vi "Get DataPoint Example.vi"() -> ()   [LabVIEW 2019]
uses:
  C:/Users/tim/Documents/kSAComm LabView Sample/kSACommInterface.dll
  kSACommInterface.dll
panel:
  out "LastError":string
  out "Connect Status":bool
  in  "IP":string="192.168.0.169"
  out "Data Point Value":string
  in  "Exit":bool
  in  "Get Data Point":bool
  # "This VI will connect with the kSA application running on the PC with the following IP Address:"
  # "Pressing this button will initiate a read of the DataPoint ColumnID from the kSA application."
  # "Pressing \"Exit\" will cleanly disconnect from the kSA application and quit the VI."
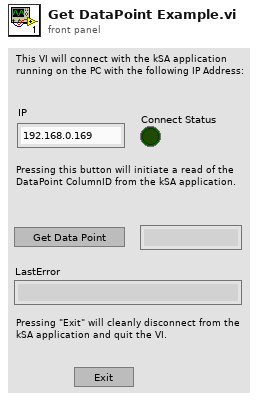
[diagram p1: front panel]
types:
  T1 = cluster{"name":string, "id":u32, "precision":i32}
  T2 = cluster{"name":string, "id":u32, "precision":i32}[]
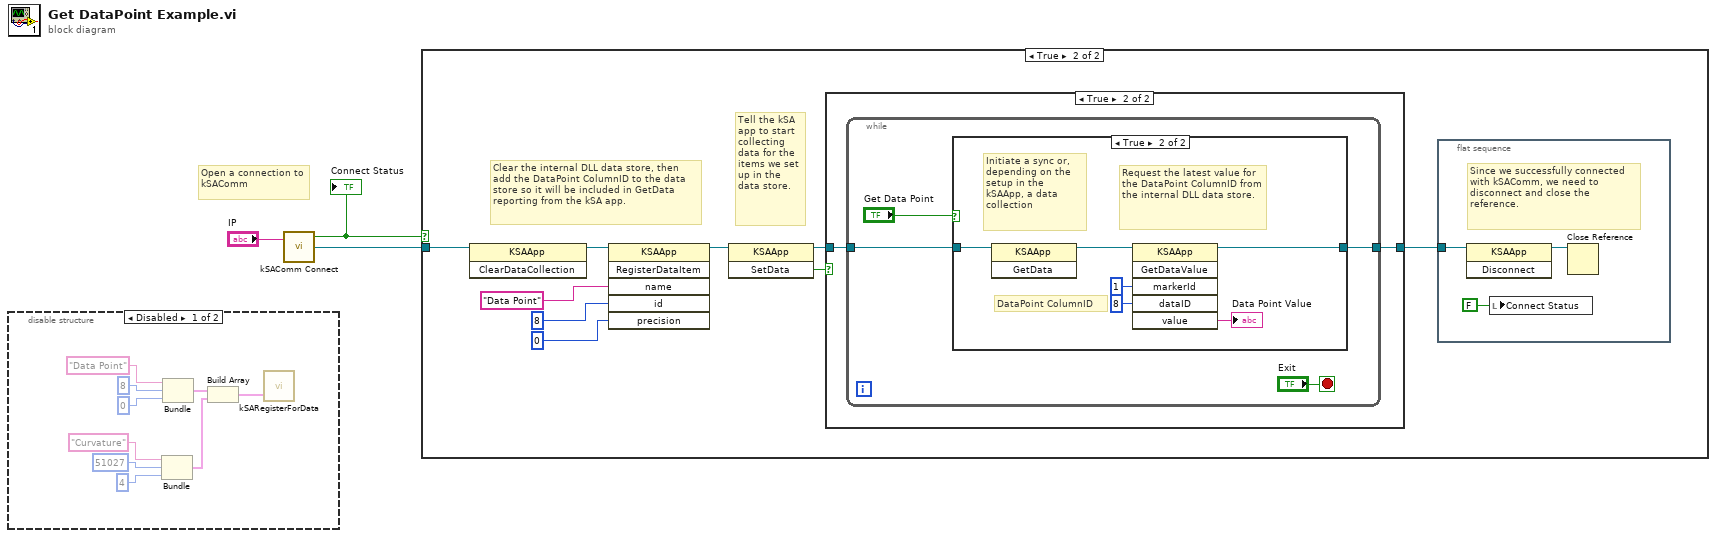
[diagram p0: block diagram]
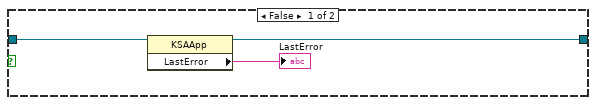
[diagram p4: hidden frame]
diagram:
  # "Open a connection to kSAComm"
  n1 = disable-structure shown="Disabled" {
    frame Disabled {
      n2 = Bundle("name"="Curvature", "id"=u32 51027, "precision"=4) -> (w4:T1)  [unwired: 1 in]
      n3 = Bundle("name"="Data Point", "id"=u32 8, "precision"=0) -> (w9:T1)  [unwired: 1 in]
      n4 = Build Array(w9, w4) -> (w8:T2)
      n5 = call "kSARegisterForData.vi"("Data Definitions"=w8) -> ()  [unwired: 1 in, 2 out]
    }
    frame Enabled {
    }
  }
  n6 = call "kSAComm Connect.vi"("IP Address"="IP") -> ("Connect"=w3:bool, "kSAComm ref out"=w1:refnum<k24>)  [unwired: 2 in]
  "Connect Status" <- w3
  n7 = case shown="True" w3 {
    tunnel: w1 -> [_ w14]
    frame False {
    }
    frame True {
      # "Tell the kSA app to start collecting data for the items we set up in the data store."
      # "Clear the internal DLL data store, then add the DataPoint ColumnID to the data store so it will be included in GetData reporting from the kSA app."
      n8 = invoke class="KSAApp" method="ClearDataCollection"(reference=w14) -> (reference out=w20:refnum<k24>)  [unwired: 2 in, 2 out]
      n9 = invoke class="KSAApp" method="RegisterDataItem"(reference=w20, "name"="Data Point", "id"=u32 8, "precision"=0) -> (reference out=w19:refnum<k24>)  [unwired: 2 in, 5 out]
      n10 = invoke class="KSAApp" method="SetData"(reference=w19) -> (reference out=w15:refnum<k24>, "SetData"=w13:bool)  [unwired: 2 in, 1 out]
      n11 = case shown="True" w13 {
        tunnel: [w22 w25] -> w21
        tunnel: w15 -> [w24 w26]
        frame False {
          n12 = property class="KSAApp"(reference=w24) -> (reference out=w22:refnum<k24>, "LastError"=→"LastError":string)  [unwired: 1 in, 1 out]
        }
        frame True {
          n13 = while {
            tunnel: w26 -> [w29]
            tunnel: [w28] -> w25
            stop <- "Exit" stop-if-true
            n14 = case shown="True" "Get Data Point" {
              tunnel: w29 -> [w31 w37]
              tunnel: [w31 w33] -> w28
              frame False {
              }
              frame True {
                # "Request the latest value for the DataPoint ColumnID from the internal DLL data store."
                # "Initiate a sync or, depending on the setup in the kSAApp, a data collection"
                # "DataPoint ColumnID"
                n15 = invoke class="KSAApp" method="GetData"(reference=w37) -> (reference out=w32:refnum<k24>)  [unwired: 2 in, 2 out]
                n16 = invoke class="KSAApp" method="GetDataValue"(reference=w32, "markerId"=u32 1, "dataID"=u32 8) -> (reference out=w33:refnum<k24>, "value"=→"Data Point Value":string)  [unwired: 3 in, 4 out]
              }
            }
          }
        }
      }
      n17 = flat-sequence {
        tunnel: w21 -> [w39]
        frame #0 {
          # "Since we successfully connected with kSAComm, we need to disconnect and close the reference."
          n18 = invoke class="KSAApp" method="Disconnect"(reference=w39) -> (reference out=w40:refnum<k24>)  [unwired: 2 in, 2 out]
          n19 = local write "Connect Status"(FALSE ("Connect")) -> ()
          n20 = Close Reference(reference=w40) -> ()  [unwired: 1 in, 1 out]
        }
      }
    }
  }
